vi "Init.vi"(8 "error in (no error)":errorcluster, 11 "Doña Rata Actor in":refnum<class "Doña Rata Actor.lvclass">) -> (0 "error out":errorcluster, 3 "Doña Rata Actor out":refnum<class "Doña Rata Actor.lvclass">)   [LabVIEW 2020, in "Doña Rata Actor.lvlib" / "Doña Rata Actor.lvclass"]
uses:
  <vilib>/Utility/config.llb/Read Key (String).vi
  <vilib>/Utility/config.llb/NI_LVConfig.lvlib
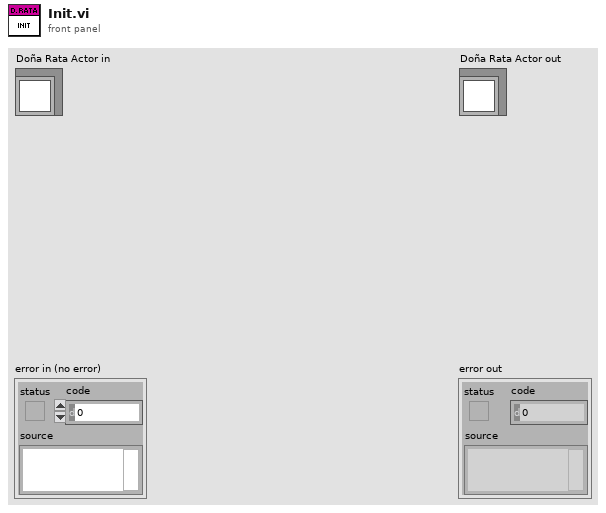
[diagram p1: front panel]
types:
  T1 = typedef "NI_LVConfig.lvlib/Config Data RefNum.ctl" = refnum<k1>
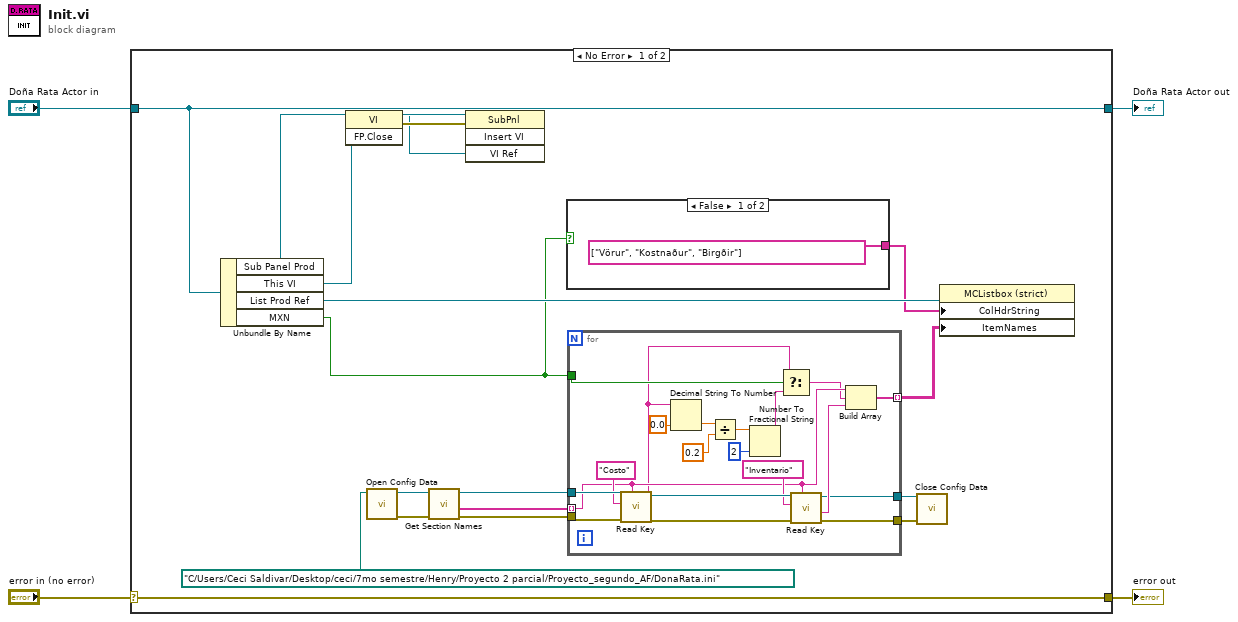
[diagram p0: block diagram]
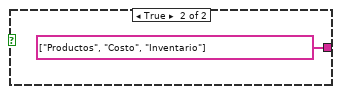
[diagram p2: hidden frame]
diagram:
  n1 = case shown="No Error" "error in (no error)" {
    selector: "error in (no error)" -> [w22 w46]
    tunnel: [w22 w46] -> w3
    tunnel: [w18 w45] -> w1
    tunnel: "Doña Rata Actor in" -> [w18 w45]
    frame No Error {
      n2 = Unbundle By Name(w18) -> ("Sub Panel Prod"=w21:refnum<vi>, "This VI"=w20:refnum<vi>, "List Prod Ref"=w9:refnum<vi>, "MXN"=w5:bool)
      n3 = invoke class="VI" method="FP.Close"(reference=w20) -> (reference out=w6:refnum<vi>, error out=w19:errorcluster)  [unwired: 2 in, 1 out]
      n4 = call <vilib>:"Open Config Data.vi"("configuration file path"=path "C:/Users/Ceci Saldivar/Desktop/ceci/7mo semestre/Henry/Proyecto 2 parcial/Proyecto_segundo_AF/DonaRata.ini") -> ("error out"=w15:errorcluster, "refnum"=w16:T1)  [unwired: 8 in, 1 out]
      n5 = call <vilib>:"Get Section Names.vi"("error in (no error)"=w15, "refnum"=w16) -> ("error out"=w13:errorcluster, "section names"=w12:string[], "refnum out"=w14:T1)  [unwired: 7 in]
      n6 = invoke class="SubPnl" method="Insert VI"(reference=w21, error in=w19, "VI Ref"=w6) -> ()  [unwired: 1 in, 4 out]
      n7 = case shown="False" w5 {
        tunnel: [string[] ["Vörur", "Kostnaður", "Birgðir"] ("Column Header Strings[]") string[] ["Productos", "Costo", "Inventario"] ("Column Header Strings[]")] -> w8
        frame False {
        }
        frame True {
        }
      }
      n8 = for {
        tunnel: w14 -> [w44]
        tunnel: w13 -> [w39]
        tunnel: w12 -> [w38] mode=indexing
        tunnel: [w36] -> w11
        tunnel: [w35] -> w10
        tunnel: [w34] -> w7 mode=indexing
        tunnel: w5 -> [w33]
        n9 = call-poly <vilib>:"Read Key.vi"("section"=w38, "error in (no error)"=w39, "key"="Costo", "refnum"=w44) -> ("error out"=w40:errorcluster, "value"=w32:string, "refnum out"=w42:T1)  [unwired: 4 in, 1 out]
        n10 = Decimal String To Number(string=w32, default (0L)=0.0) -> (number=w30:dbl)  [unwired: 1 in, 1 out]
        n11 = Divide(x=w30, y=0.2) -> (x/y=w28:dbl)
        n12 = Number To Fractional String(number=w28, precision (6)=i16 2) -> (F-format string=w26:string)  [unwired: 2 in]
        n13 = Select(t=w32, s=w33, f=w26) -> (s? t:f=w25:string)
        n14 = call-poly <vilib>:"Read Key.vi"("section"=w38, "error in (no error)"=w40, "key"="Inventario", "refnum"=w42) -> ("error out"=w35:errorcluster, "value"=w37:string, "refnum out"=w36:T1)  [unwired: 4 in, 1 out]
        n15 = Build Array(w38, w25, w37) -> (w34:string[])
      }
      n16 = call <vilib>:"Close Config Data.vi"("error in (no error)"=w10, "refnum"=w11) -> ()  [unwired: 8 in, 2 out]
      n17 = property class="MCListbox (strict)"(reference=w9, "ColHdrString"=w8, "ItemNames"=w7) -> ()  [unwired: 1 in, 2 out]
    }
    frame Error {
    }
  }
  "error out" <- w3
  "Doña Rata Actor out" <- w1
